vi "Get Current Temperature.vi"(8 "error in (no error)":cluster{"状态":bool, "代码":i32, "源":string} caption="错误输入（无错误）", 11 "仿真蒸发冷却器":refnum<class "Simulated Evaporative Cooler.lvclass">) -> (0 "error out":cluster{"状态":bool, "代码":i32, "源":string} caption="错误输出", 2 "水位":dbl)   [LabVIEW 2015, in "Simulated Evaporative Cooler.lvclass"]
doc: "该VI读取当前室内空气温度。"
uses:
  Simulated Evaporative Cooler.lvclass
  Simulation Data_Global.vi
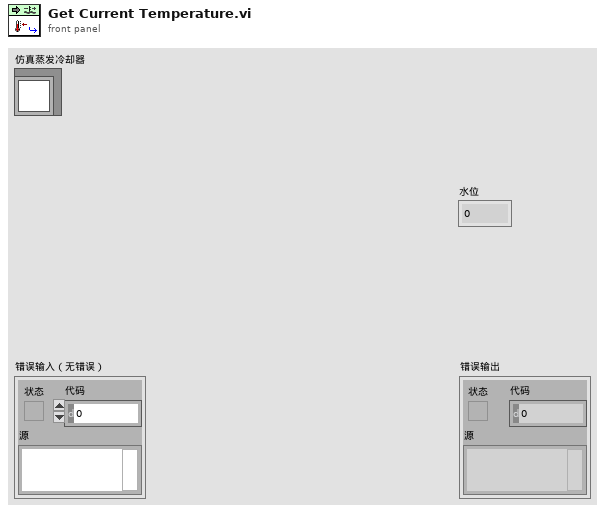
[diagram p1: front panel]
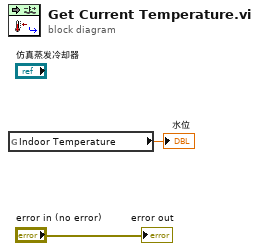
[diagram p0: block diagram]
diagram:
  n1 = global read "Simulation Data_Global.vi" "Indoor Temperature"() -> (→"水位":dbl)
  "error out" <- "error in (no error)"
